vi "JKI State Machine C.vi"() -> ()   [LabVIEW 2020]
uses:
  _JKISMQFGV.vi
  JKI-State-Machine-Plus.lvlib
panel:
  out "Name":string[](array[string])
  out "String Cache":string
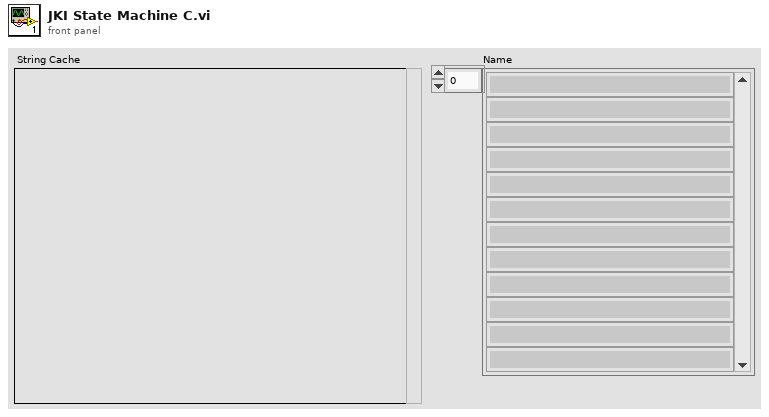
[diagram p1: front panel]
types:
  T1 = enum32{"Invalid", "Standard", "Closed", "Hidden", "Minimized", "Maximized"}
  T2 = enum32{"invalid app kind", "Development System", "Run Time System", "Student Edition", "Embedded LabVIEW", "Evaluation", "Custom"}
  T3 = cluster{"Core":cluster{"Current VI Reference":refnum<vi>, "Close Panel on Exit?":bool}, "Your Boolean data":bool, "Your string data":string}
  T4 = cluster{"Current VI Reference":refnum<vi>, "Close Panel on Exit?":bool}
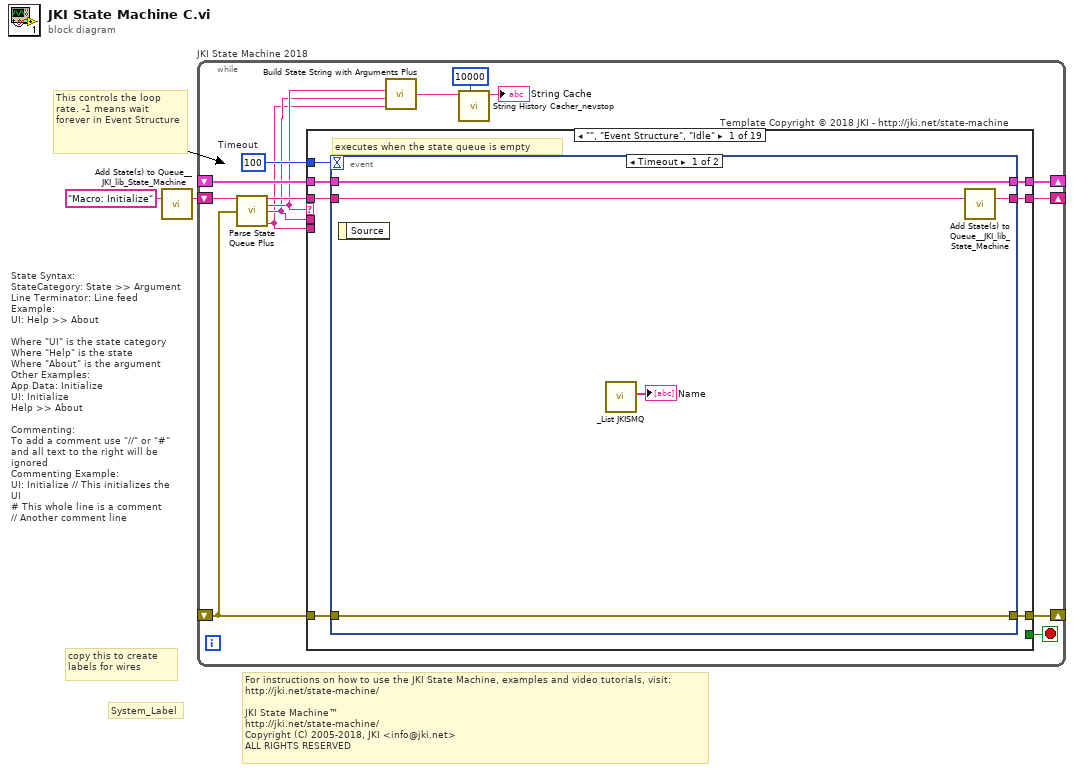
[diagram p0: block diagram]
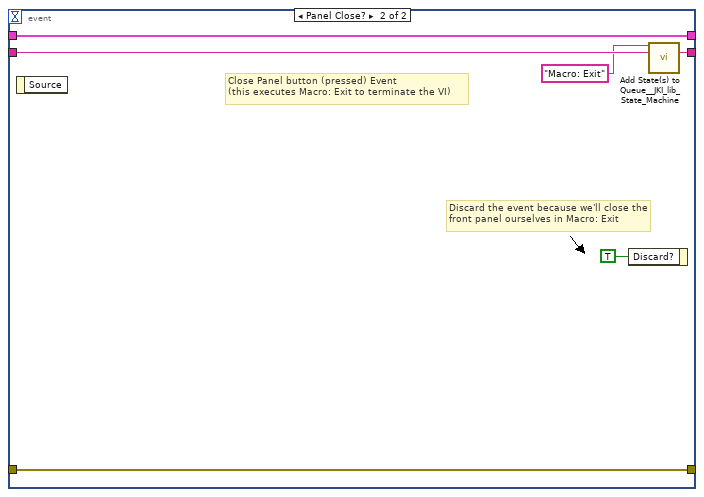
[diagram p2: hidden frame]
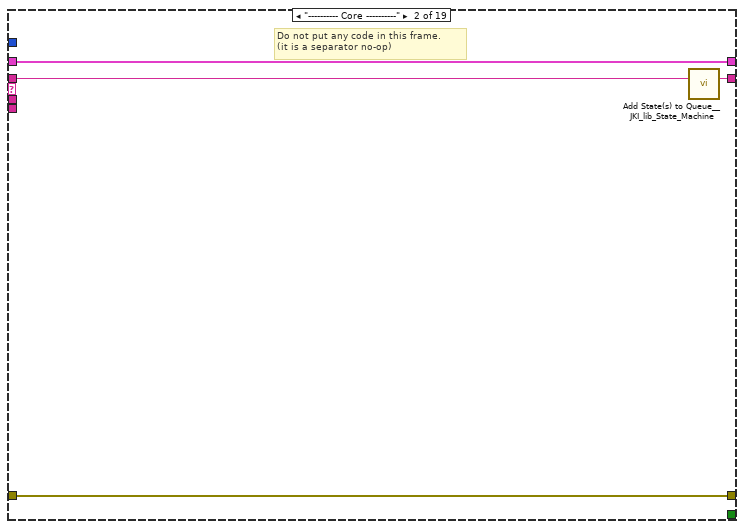
[diagram p3: hidden frame]
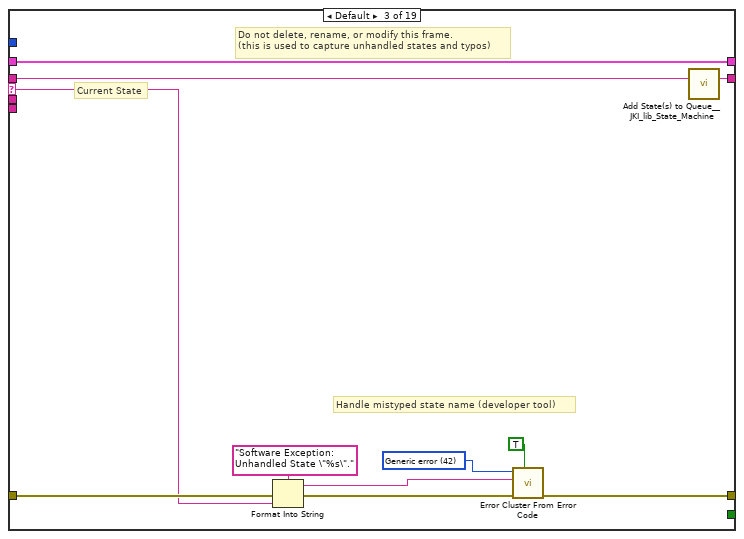
[diagram p4: hidden frame]
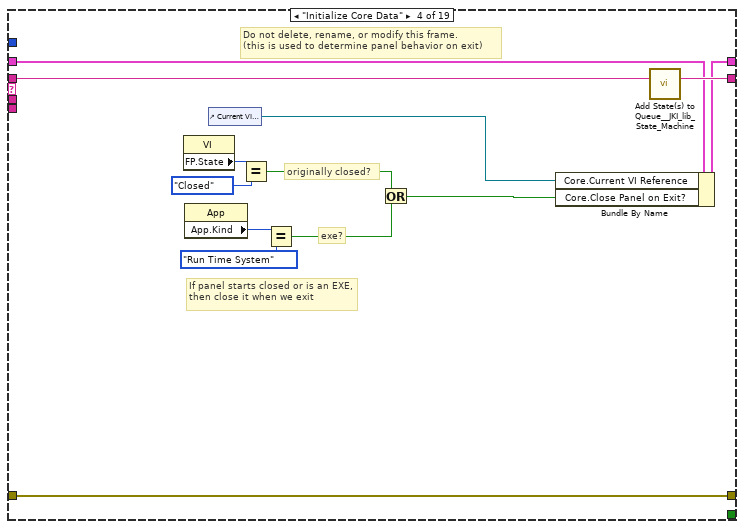
[diagram p5: hidden frame]
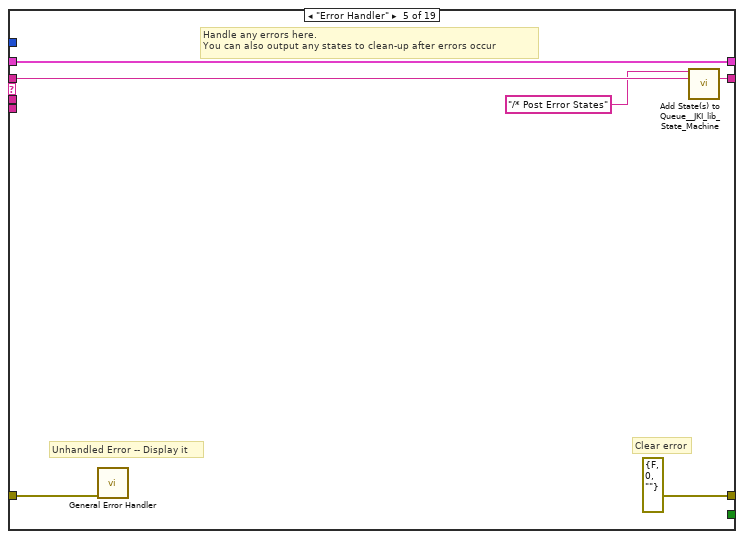
[diagram p6: hidden frame]
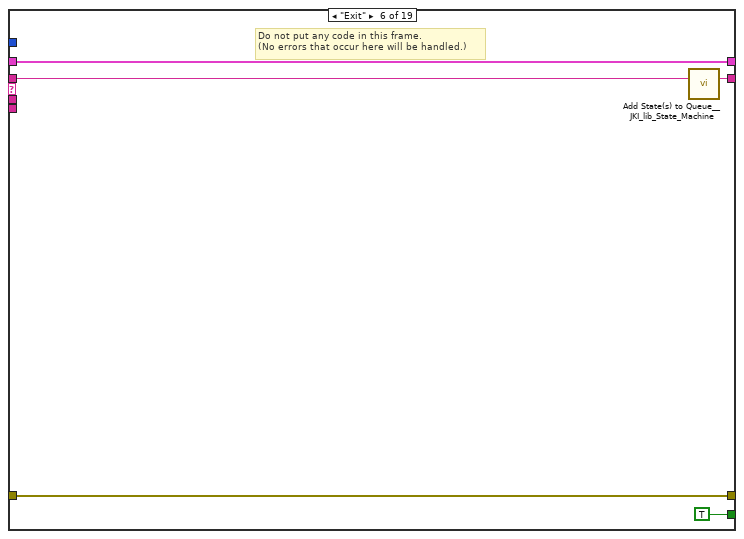
[diagram p7: hidden frame]
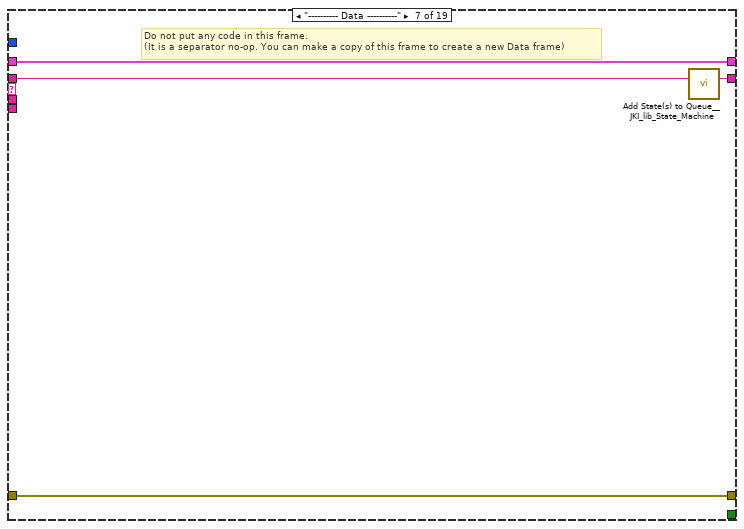
[diagram p8: hidden frame]
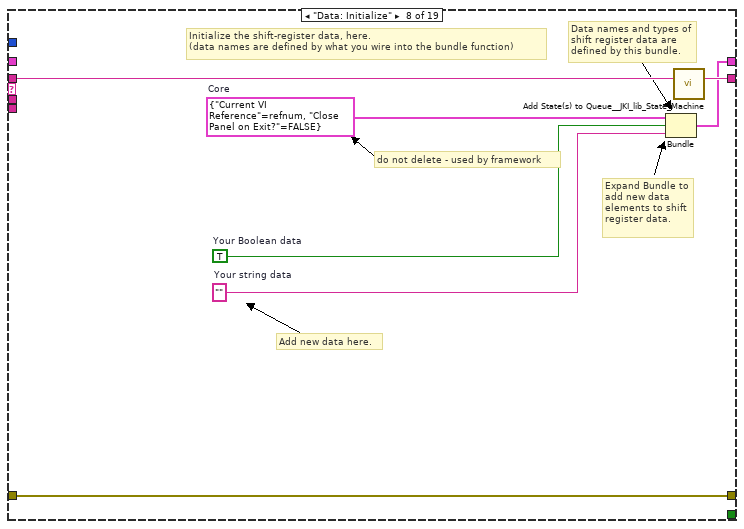
[diagram p9: hidden frame]
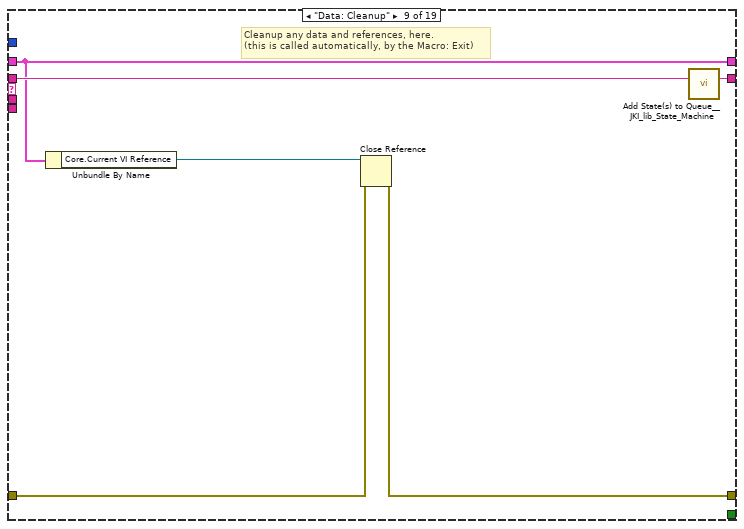
[diagram p10: hidden frame]
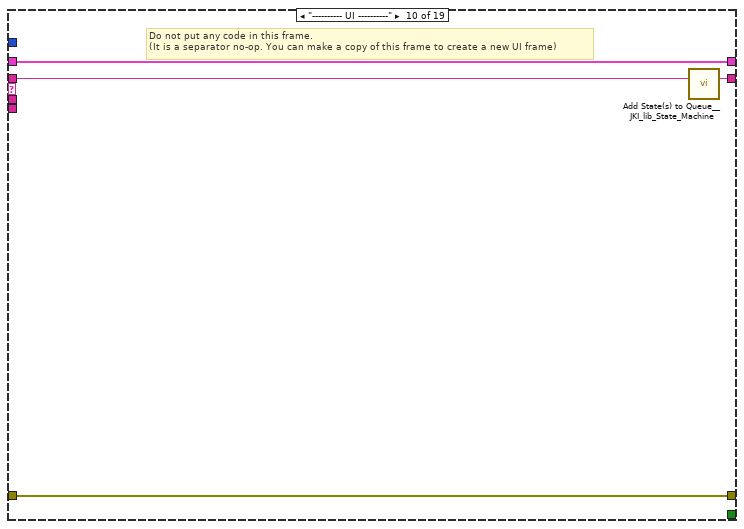
[diagram p11: hidden frame]
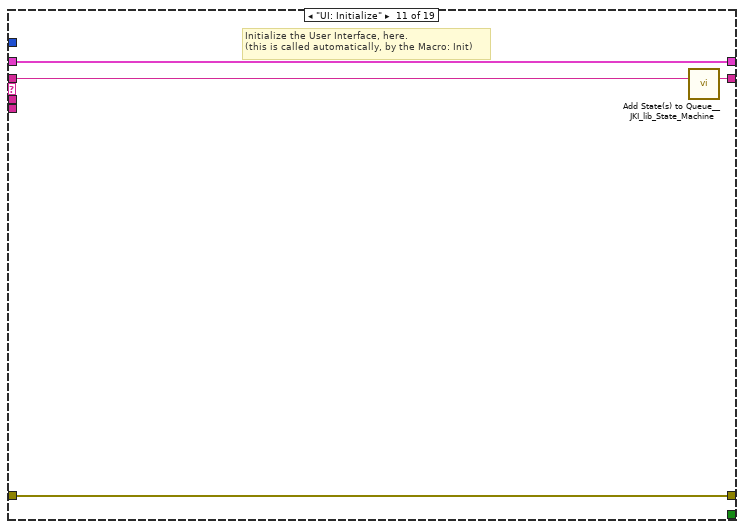
[diagram p12: hidden frame]
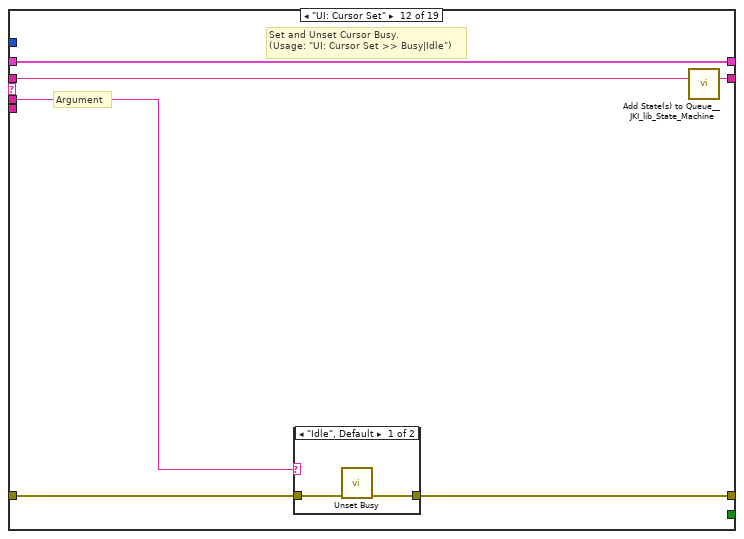
[diagram p13: hidden frame]
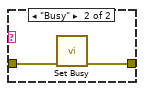
[diagram p14: hidden frame]
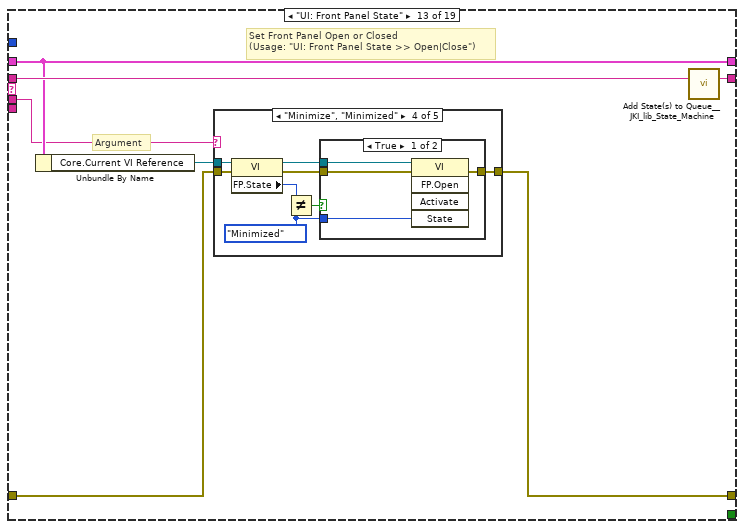
[diagram p15: hidden frame]
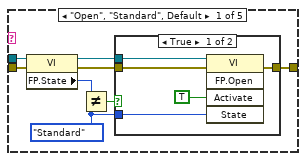
[diagram p16: hidden frame]
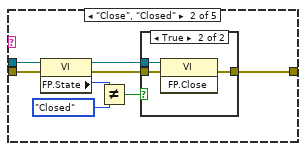
[diagram p18: hidden frame]
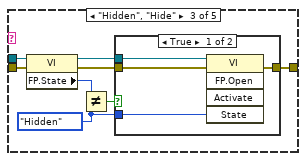
[diagram p20: hidden frame]
diagram:
  # "For instructions on how to use the JKI State Machine, examples and video tutorials, visit:\nhttp://jki.net/state-machine/\n\nJKI State Machine™\nhttp://jki.net/state-machine/\nCopyright (C) 2005-2018, JKI <info@jki.net>\nALL RIGHTS RESERVED"
  # "State Syntax:\nStateCategory: State >> Argument\nLine Terminator: Line feed\nExample:\nUI: Help >> About\n\nWhere \"UI\" is the state category\nWhere \"Help\" is the state\nWhere \"About\" is the argument\nOther Examples:\nApp Data: Initialize\nUI: Initialize\nHelp >> About\n\nCommenting:\nTo add a comment use \"//\" or \"#\" and all text to the right will be ignored\nCommenting Example:\nUI: Initialize // This initializes the UI\n# This whole line is a comment\n// Another comment line"
  # "copy this to create labels for wires"
  # "This controls the loop rate. -1 means wait forever in Event Structure"
  # "System_Label"
  n1 = call <vilib>:"Add State(s) to Queue__JKI_lib_State_Machine.vi"("State(s) in (\"\")"="Macro: Initialize") -> ("States Out"=w2:string)  [unwired: 14 in]
  n2 = while "JKI State Machine 2018" {
    shift-right: [w12] -> _
    shift-left: _ -> [w11]
    shift-right: [w15] -> _
    shift-left: _ -> [w9]
    shift-right: [w14] -> _
    shift-left: w2 -> [w16]
    stop <- w13 stop-if-true
    w10 = 100  # Timeout
    # "Template Copyright © 2018 JKI - http://jki.net/state-machine"
    n3 = call "Parse State Queue Plus.vi"("State Queue"=w16, "Error In (no error)"=w9) -> ("Remaining States"=w17:string, "Current State"=w7:string, "Arguments"=w6:string, "From Who"=w5:string)  [unwired: 10 in]
    n4 = case shown="\"\", \"Event Structure\", \"Idle\"" w7 {
      selector: w7 -> [_ _ w40 _ _ _ _ _ _ _ _ _ _ _ _ _ _ _ _]
      tunnel: w17 -> [w24 w39 w44 w63 w69 w74 w78 w85 w91 w95 w99 w105 w116 w185 w190 w200 w204 w208 w212]
      tunnel: w6 -> [_ _ _ _ _ _ _ _ _ _ _ w100 w110 _ _ _ _ _ _]
      tunnel: w11 -> [w22 w36 w42 w56 w66 w72 w75 _ w86 w92 w97 w103 w112 w182 w187 w197 w201 w205 w209]
      tunnel: [w21 w37 w46 w60 errorcluster {"status"=FALSE, "code"=0, "source"=""} ("error out") w71 w76 w82 w87 w93 w96 w101 w113 w183 w188 w198 w202 w206 w210] -> w15
      tunnel: w9 -> [w20 w37 w45 w60 w65 w71 w76 w82 w88 w93 w96 w102 w114 w183 w188 w198 w202 w206 w210]
      tunnel: [w23 w38 w43 w62 w68 w73 w77 w84 w90 w94 w98 w104 w115 w184 w189 w199 w203 w207 w211] -> w14
      tunnel: [_ _ _ _ _ TRUE _ _ _ _ _ _ _ _ _ _ _ _ _] -> w13
      tunnel: [w19 w36 w42 w61 w66 w72 w75 w83 w86 w92 w97 w103 w112 w182 w187 w197 w201 w205 w209] -> w12
      tunnel: w10 -> [w18 _ _ _ _ _ _ _ _ _ _ _ _ _ _ _ _ _ _]
      tunnel: w5 -> [_ _ _ _ _ _ _ _ _ _ _ _ _ _ _ _ _ _ _]
      frame "", "Event Structure", "Idle" {
        # "executes when the state queue is empty"
        n5 = event shown="[0] Timeout" {
          selector: _ -> [_ _]
          dyn-events: _ -> [_ _]
          timeout: w18 -> [_ _]
          tunnel: w24 -> [w29 w35]
          tunnel: [w28 w34] -> w23
          tunnel: w22 -> [w26 w32]
          tunnel: [w27 w33] -> w21
          tunnel: w20 -> [w27 w33]
          tunnel: [w26 w32] -> w19
          event Timeout {
            n6 = event-data() -> ()  [unwired: 1 in, 1 out]
            n7 = call "_List JKISMQ.vi"() -> ("Name"=→"Name":string[])  [unwired: 9 in, 2 out]
            n8 = call <vilib>:"Add State(s) to Queue__JKI_lib_State_Machine.vi"("State(s) in (\"\")"=w29) -> ("States Out"=w28:string)  [unwired: 14 in]
          }
          event Panel Close? {
            # "Discard the event because we'll close the front panel ourselves in Macro: Exit"
            # "Close Panel button (pressed) Event\n(this executes Macro: Exit to terminate the VI)"
            n9 = event-data() -> ()  [unwired: 1 in, 1 out]
            n10 = event-data("Discard?"=TRUE) -> ()  [unwired: 1 in, 1 out]
            n11 = call <vilib>:"Add State(s) to Queue__JKI_lib_State_Machine.vi"("State(s) in Front (\"\")"="Macro: Exit", "State(s) in (\"\")"=w35) -> ("States Out"=w34:string)  [unwired: 13 in]
          }
        }
      }
      frame "---------- Core ----------" {
        # "Do not put any code in this frame.\n(it is a separator no-op)"
        n12 = call <vilib>:"Add State(s) to Queue__JKI_lib_State_Machine.vi"("State(s) in (\"\")"=w39) -> ("States Out"=w38:string)  [unwired: 14 in]
      }
      frame Default {
        w49 = 42 items=["No error", "Argument error", "Memory is full", "Out of zone", "End of file", "File already open", "Generic file I/O error", "File not found", "File permission error", "Disk is full", "Duplicate path", "Too many files open", "System feature not enabled", "Resource file not found", "Cannot add resource", "Resource not found", "Image not found", "Image memory error", "Pen does not exist", "Config type invalid", "Config token not found", "Config parse error", "Config memory error", "Bad external code format", "Bad external code offset", "External code not present", "Null window", "Destroy window error", "Null menu", "Print aborted", "Bad print record", "Print driver error", "Windows error during printing", "Memory error during printing", "Print dialog error", "Generic print error", "Invalid device refnum", "Device not found", "Device parameter error", "Device unit error", "Cannot open device", "Device call aborted", "Generic error", "Cancelled by user", "Object ID too low", "Object ID too high", "Object not in heap", "Unknown heap", "Unknown object (invalid DefProc)", "Unknown object (DefProc not in table)", "Message out of range", "Invalid (null) method", "Unknown message", "Manager call not supported", "Bad address", "Network operation in progress", "Network operation timed out", "Connection is busy", "Network attribute not supported", "Network error", "Address in use", "System out of memory", "Connection aborted", "Connection refused", "Not connected", "Already connected", "Connection closed", "Initialization error (interapplication manager)", "Bad occurrence", "Wait on unbound occurrence handler", "Occurrence queue overflow", "Datalog type conflict", "Unused", "Unrecognized type (interapplication manager)", "Memory corrupt", "Failed to make temporary DLL", "Old CIN version", "Drag socket not found", "Failed to load drop-object", "Failed to register OLE object", "Failed to release OLE object", "Format specifier type mismatch", "Unknown format specifier", "Too few format specifiers", "Too many format specifiers", "Scan failed", "Newer CIN version", "Error converting to variant", "Runtime menu error", "Password tampered", "Variant attribute not found", "Incompatible variant data type", "Event data is not available", "Event Store is not present", "Occurrence is not found", "Event Queue is not created", "Event info is not available", "Refnum passed is NULL", "Error retrieving Class GUID", "Error retrieving CoClass GUID", "Error retrieving TypeLib GUID.", "Bad built application magic bytes.", "Specific driver is different from the specific driver associated with the Logical Name.", "There is no session opened to the class driver.", "Max Error", "MAX - Error with config objects", "MAX - Error loading configuration", "MAX - Group not supported"]
        # "Current State"
        # "Do not delete, rename, or modify this frame.\n(this is used to capture unhandled states and typos)"
        # "Handle mistyped state name (developer tool)"
        n13 = Format Into String(format string="Software Exception: Unhandled State \"%s\"." ("message"), error in=w45, w40) -> (resulting string=w48:string, error out=w47:errorcluster)  [unwired: 1 in]
        n14 = call <vilib>:"Error Cluster From Error Code.vi"("show call chain? (False)"=TRUE, "error in (no error)"=w47, "error message (\"\")"=w48, "error code (0)"=w49) -> ("error out"=w46:errorcluster)  [unwired: 5 in]
        n15 = call <vilib>:"Add State(s) to Queue__JKI_lib_State_Machine.vi"("State(s) in (\"\")"=w44) -> ("States Out"=w43:string)  [unwired: 14 in]
      }
      frame "Initialize Core Data" {
        # "Do not delete, rename, or modify this frame.\n(this is used to determine panel behavior on exit)"
        # "originally closed?"
        # "exe?"
        # "If panel starts closed or is an EXE, then close it when we exit"
        n16 = property class="VI"() -> ("FP.State"=w53:T1)  [unwired: 2 in, 2 out]
        n17 = property class="App"() -> ("App.Kind"=w59:T2)  [unwired: 2 in, 2 out]
        n18 = control-ref of="Current VI Reference"() -> (w54:refnum<vi>)
        n19 = Equal?(x=w53, y=T1."Closed" ("Front Panel Window:State")) -> (x = y?=w51:bool)
        n20 = Equal?(x=w59, y=T2."Run Time System" ("Application:Kind")) -> (x = y?=w57:bool)
        n21 = Or(x=w51, y=w57) -> (x .or. y?=w55:bool)
        n22 = Bundle By Name(cluster=w56, "Core.Current VI Reference"=w54, "Core.Close Panel on Exit?"=w55) -> (w61:T3)
        n23 = call <vilib>:"Add State(s) to Queue__JKI_lib_State_Machine.vi"("State(s) in (\"\")"=w63) -> ("States Out"=w62:string)  [unwired: 14 in]
      }
      frame "Error Handler" {
        # "Unhandled Error -- Display it"
        # "Handle any errors here.\nYou can also output any states to clean-up after errors occur"
        # "Clear error"
        n24 = call <vilib>:"General Error Handler.vi"("error in (no error)"=w65) -> ()  [unwired: 10 in, 5 out]
        n25 = call <vilib>:"Add State(s) to Queue__JKI_lib_State_Machine.vi"("State(s) in Front (\"\")"="/* Post Error States", "State(s) in (\"\")"=w69) -> ("States Out"=w68:string)  [unwired: 13 in]
      }
      frame "Exit" {
        # "Do not put any code in this frame.\n(No errors that occur here will be handled.)"
        n26 = call <vilib>:"Add State(s) to Queue__JKI_lib_State_Machine.vi"("State(s) in (\"\")"=w74) -> ("States Out"=w73:string)  [unwired: 14 in]
      }
      frame "---------- Data ----------" {
        # "Do not put any code in this frame.\n(It is a separator no-op. You can make a copy of this frame to create a new Data frame)"
        n27 = call <vilib>:"Add State(s) to Queue__JKI_lib_State_Machine.vi"("State(s) in (\"\")"=w78) -> ("States Out"=w77:string)  [unwired: 14 in]
      }
      frame "Data: Initialize" {
        w79 = T4 {"Current VI Reference"=refnum, "Close Panel on Exit?"=FALSE}  # Core
        w81 = TRUE  # Your Boolean data
        w80 = ""  # Your string data
        # "do not delete - used by framework"
        # "Expand Bundle to add new data elements to shift register data."
        # "Add new data here."
        # "Data names and types of shift register data are defined by this bundle."
        # "Initialize the shift-register data, here.\n(data names are defined by what you wire into the bundle function)"
        n28 = Bundle("Core"=w79, "Your Boolean data"=w81, "Your string data"=w80) -> (w83:T3)  [unwired: 1 in]
        n29 = call <vilib>:"Add State(s) to Queue__JKI_lib_State_Machine.vi"("State(s) in (\"\")"=w85) -> ("States Out"=w84:string)  [unwired: 14 in]
      }
      frame "Data: Cleanup" {
        # "Cleanup any data and references, here.\n(this is called automatically, by the Macro: Exit)"
        n30 = Unbundle By Name(w86) -> ("Core.Current VI Reference"=w89:refnum<vi>)
        n31 = Close Reference(reference=w89, error in (no error)=w88) -> (error out=w87:errorcluster)
        n32 = call <vilib>:"Add State(s) to Queue__JKI_lib_State_Machine.vi"("State(s) in (\"\")"=w91) -> ("States Out"=w90:string)  [unwired: 14 in]
      }
      frame "---------- UI ----------" {
        # "Do not put any code in this frame.\n(It is a separator no-op. You can make a copy of this frame to create a new UI frame)"
        n33 = call <vilib>:"Add State(s) to Queue__JKI_lib_State_Machine.vi"("State(s) in (\"\")"=w95) -> ("States Out"=w94:string)  [unwired: 14 in]
      }
      frame "UI: Initialize" {
        # "Initialize the User Interface, here.\n(this is called automatically, by the Macro: Init)"
        n34 = call <vilib>:"Add State(s) to Queue__JKI_lib_State_Machine.vi"("State(s) in (\"\")"=w99) -> ("States Out"=w98:string)  [unwired: 14 in]
      }
      frame "UI: Cursor Set" {
        # "Argument"
        # "Set and Unset Cursor Busy.\n(Usage: \"UI: Cursor Set >> Busy|Idle\")"
        n35 = case shown="\"Idle\", Default" w100 {
          tunnel: w102 -> [w107 w109]
          tunnel: [w106 w108] -> w101
          frame "Idle", Default {
            n36 = call <vilib>:"Unset Busy.vi"("error in (no error)"=w107) -> ("error out"=w106:errorcluster)  [unwired: 10 in]
          }
          frame "Busy" {
            n37 = call <vilib>:"Set Busy.vi"("error in (no error)"=w109) -> ("error out"=w108:errorcluster)  [unwired: 9 in, 1 out]
          }
        }
        n38 = call <vilib>:"Add State(s) to Queue__JKI_lib_State_Machine.vi"("State(s) in (\"\")"=w105) -> ("States Out"=w104:string)  [unwired: 14 in]
      }
      frame "UI: Front Panel State" {
        # "Argument"
        # "Set Front Panel Open or Closed\n(Usage: \"UI: Front Panel State >> Open|Close\")"
        n39 = Unbundle By Name(w112) -> ("Core.Current VI Reference"=w111:refnum<vi>)
        n40 = case shown="\"Minimize\", \"Minimized\"" w110 {
          tunnel: w114 -> [w122 w137 w148 w161 w174]
          tunnel: [w124 w138 w150 w163 w176] -> w113
          tunnel: w111 -> [w123 w135 w149 w162 w175]
          frame "Open", "Standard", Default {
            w117 = T1."Standard" ("State")
            n41 = property class="VI"(reference=w123, error in=w122) -> (reference out=w120:refnum<vi>, error out=w121:errorcluster, "FP.State"=w119:T1)
            n42 = Not Equal?(x=w119, y=w117) -> (x != y?=w118:bool)
            n43 = case shown="True" w118 {
              tunnel: [w128 w130] -> w124
              tunnel: w121 -> [w127 w130]
              tunnel: w120 -> [w126 _]
              tunnel: w117 -> [w125 _]
              frame True {
                n44 = invoke class="VI" method="FP.Open"(reference=w126, error in=w127, "Activate"=TRUE, "State"=w125) -> (error out=w128:errorcluster)  [unwired: 1 in, 4 out]
              }
              frame False {
              }
            }
          }
          frame "Close", "Closed" {
            n45 = property class="VI"(reference=w135, error in=w137) -> (reference out=w134:refnum<vi>, error out=w136:errorcluster, "FP.State"=w132:T1)
            n46 = Not Equal?(x=w132, y=T1."Closed" ("Front Panel Window:State")) -> (x != y?=w131:bool)
            n47 = case shown="True" w131 {
              tunnel: [w139 w142] -> w138
              tunnel: w136 -> [w139 w141]
              tunnel: w134 -> [_ w140]
              frame False {
              }
              frame True {
                n48 = invoke class="VI" method="FP.Close"(reference=w140, error in=w141) -> (error out=w142:errorcluster)  [unwired: 1 in, 2 out]
              }
            }
          }
          frame "Hidden", "Hide" {
            w143 = T1."Hidden" ("State")
            n49 = property class="VI"(reference=w149, error in=w148) -> (reference out=w146:refnum<vi>, error out=w147:errorcluster, "FP.State"=w145:T1)
            n50 = Not Equal?(x=w145, y=w143) -> (x != y?=w144:bool)
            n51 = case shown="True" w144 {
              tunnel: [w154 w155] -> w150
              tunnel: w147 -> [w153 w155]
              tunnel: w146 -> [w152 _]
              tunnel: w143 -> [w151 _]
              frame True {
                n52 = invoke class="VI" method="FP.Open"(reference=w152, error in=w153, "State"=w151) -> (error out=w154:errorcluster)  [unwired: 2 in, 4 out]
              }
              frame False {
              }
            }
          }
          frame "Minimize", "Minimized" {
            w156 = T1."Minimized" ("State")
            n53 = property class="VI"(reference=w162, error in=w161) -> (reference out=w159:refnum<vi>, error out=w160:errorcluster, "FP.State"=w158:T1)
            n54 = Not Equal?(x=w158, y=w156) -> (x != y?=w157:bool)
            n55 = case shown="True" w157 {
              tunnel: [w167 w168] -> w163
              tunnel: w160 -> [w166 w168]
              tunnel: w159 -> [w165 _]
              tunnel: w156 -> [w164 _]
              frame True {
                n56 = invoke class="VI" method="FP.Open"(reference=w165, error in=w166, "State"=w164) -> (error out=w167:errorcluster)  [unwired: 2 in, 4 out]
              }
              frame False {
              }
            }
          }
          frame "Maximize", "Maximized" {
            w169 = T1."Maximized" ("State")
            n57 = property class="VI"(reference=w175, error in=w174) -> (reference out=w172:refnum<vi>, error out=w173:errorcluster, "FP.State"=w171:T1)
            n58 = Not Equal?(x=w171, y=w169) -> (x != y?=w170:bool)
            n59 = case shown="True" w170 {
              tunnel: [w180 w181] -> w176
              tunnel: w173 -> [w179 w181]
              tunnel: w172 -> [w178 _]
              tunnel: w169 -> [w177 _]
              frame True {
                n60 = invoke class="VI" method="FP.Open"(reference=w178, error in=w179, "State"=w177) -> (error out=w180:errorcluster)  [unwired: 2 in, 4 out]
              }
              frame False {
              }
            }
          }
        }
        n61 = call <vilib>:"Add State(s) to Queue__JKI_lib_State_Machine.vi"("State(s) in (\"\")"=w116) -> ("States Out"=w115:string)  [unwired: 14 in]
      }
      frame "---------- Macro ----------" {
        # "Do not put any code in this frame.\n(It is a separator no-op. You can make a copy of this frame to create a new Macro frame)"
        n62 = call <vilib>:"Add State(s) to Queue__JKI_lib_State_Machine.vi"("State(s) in (\"\")"=w185) -> ("States Out"=w184:string)  [unwired: 14 in]
      }
      frame "Macro: Initialize" {
        w186 = "Data: Initialize\nInitialize Core Data\nUI: Initialize\nUI: Front Panel State >> Open"  # Data: Initialize Initialize Core Data UI: Initialize UI: Front Panel State >> Open
        # "Initialization Macro\n(This is called once, when the VI starts)"
        n63 = call <vilib>:"Add State(s) to Queue__JKI_lib_State_Machine.vi"("State(s) in Front (\"\")"=w186, "State(s) in (\"\")"=w190) -> ("States Out"=w189:string)  [unwired: 13 in]
      }
      frame "Macro: Exit" {
        # "Exit Macro\n(This is called once, when the VI exits)"
        n64 = Unbundle By Name(w197) -> ("Core.Close Panel on Exit?"=w196:bool)
        n65 = Select(t="UI: Front Panel State >> Close", s=w196, f="") -> (s? t:f=w193:string)
        n66 = call <vilib>:"Add State(s) to Queue__JKI_lib_State_Machine.vi"("State(s) in (\"\")"=w193, "State(s) at Back (\"\")"="Data: Cleanup\nExit") -> ("States Out"=w191:string)  [unwired: 13 in]
        n67 = call <vilib>:"Add State(s) to Queue__JKI_lib_State_Machine.vi"("State(s) in Front (\"\")"=w191, "State(s) in (\"\")"=w200) -> ("States Out"=w199:string)  [unwired: 13 in]
      }
      frame "---------- New Category ----------" {
        # "Template Separator\n(You can make a copy of, or modify, this frame)"
        n68 = call <vilib>:"Add State(s) to Queue__JKI_lib_State_Machine.vi"("State(s) in (\"\")"=w204) -> ("States Out"=w203:string)  [unwired: 14 in]
      }
      frame "New Category: 1" {
        # "Your code here.\n(You can make a copy of, or modify, this frame)"
        n69 = call <vilib>:"Add State(s) to Queue__JKI_lib_State_Machine.vi"("State(s) in (\"\")"=w208) -> ("States Out"=w207:string)  [unwired: 14 in]
      }
      frame "New Category: 2" {
        # "Your code here.\n(You can make a copy of, or modify, this frame)"
        n70 = call <vilib>:"Add State(s) to Queue__JKI_lib_State_Machine.vi"("State(s) in (\"\")"=w212) -> ("States Out"=w211:string)  [unwired: 14 in]
      }
    }
    n71 = call "Build State String with Arguments Plus.vi"("Source (\"\")"=w5, "Arguments (\"\")"=w6, "State"=w7) -> ("State with Arguments"=w8:string)  [unwired: 3 in]
    n72 = call <userlib>:"String History Cacher_nevstop.vi"("length"=10000, "String"=w8) -> ("String Cache"=→"String Cache":string)  [unwired: 9 in]
  }
